vi "FTW-Actor-ConstructExtended.vi"(0 "FTW Actor Instance Type":refnum<class "FTW-ActorInstance.lvclass">, 7 "Actor Instance Configuration":string, 11 "error in":errorcluster) -> (4 "FTW Actor Instance":refnum<class "FTW-ActorInstance.lvclass">, 8 "Subscriber Registration":refnum<event-registration>, 15 "error out":errorcluster)   [LabVIEW 2015, in "FTW-ActorInstance.lvclass"]
uses:
  FTW-ActorInstance.lvclass
  Message/Base/FTW-Message.lvclass
  FTW-ActorInstance.lvclass/FTW-ActorInstance.ctl
  Connector/FTW-ActorConnector.lvclass
  Publisher/FTW-Publisher.lvclass
  Ether/FTW-Ether.lvclass
  Subscriber/FTW-Subscriber.lvclass
panel:
  # "Inputs"
  # "Outputs"
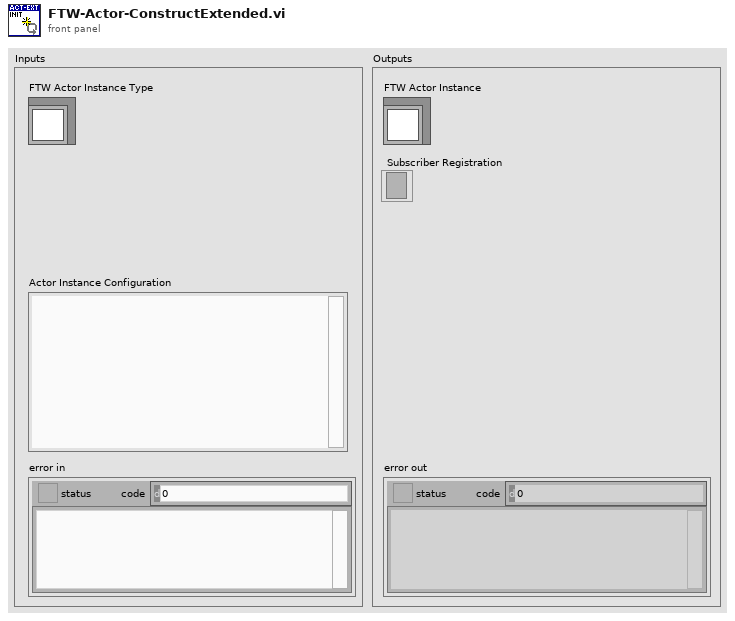
[diagram p1: front panel]
types:
  T1 = cluster{"String":string, "Fetched Address":string, "FTW Actor Connector":refnum<class "FTW-ActorConnector.lvclass">, bool}
  T2 = cluster{"String":string, "Actual Address":string, "FTW-Publisher Out":refnum<class "FTW-Publisher.lvclass">}
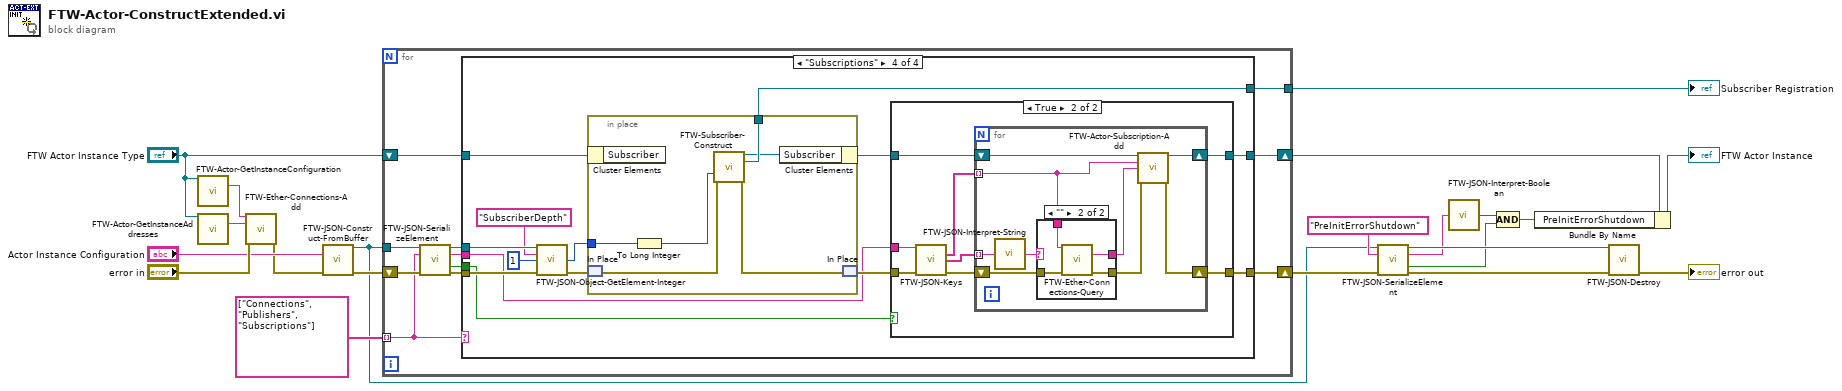
[diagram p0: block diagram]
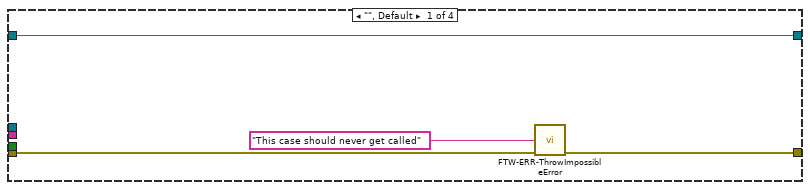
[diagram p2: hidden frame]
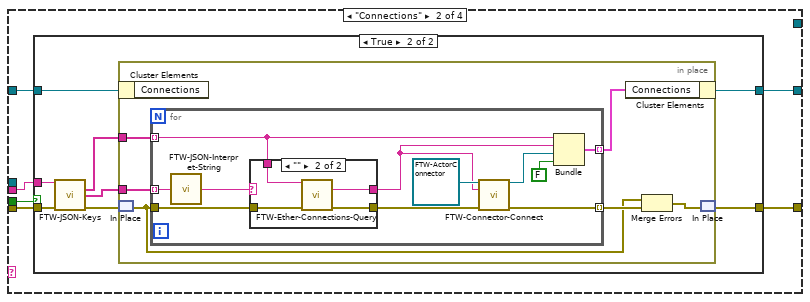
[diagram p3: hidden frame]
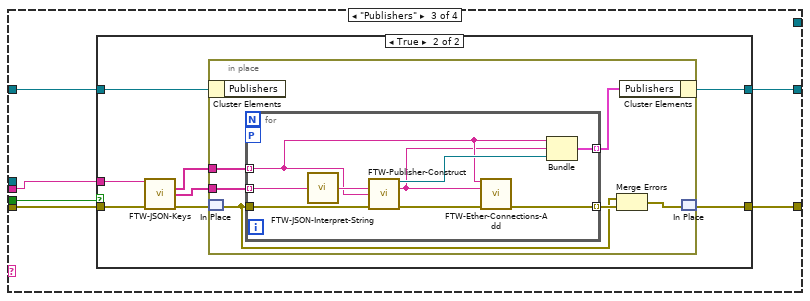
[diagram p6: hidden frame]
diagram:
  n1 = call "FTW-Actor-GetInstanceConfiguration.vi"("FTW Actor Instance"="FTW Actor Instance Type") -> ("Identity"=w4:string)  [unwired: 12 in, 2 out]
  n2 = call "FTW-Actor-GetInstanceAddresses.vi"("FTW Actor Instance"="FTW Actor Instance Type") -> ("Inbox Address"=w3:string)  [unwired: 12 in, 2 out]
  n3 = call "FTW-Ether-Connections-Add.vi"("Connection"=w4, "Address"=w3, "error in"="error in") -> ("error out"=w2:errorcluster)  [unwired: 12 in]
  n4 = call "FTW-JSON-Construct-FromBuffer.vi"("JSON String (UTF-8)"="Actor Instance Configuration", "error in"=w2) -> ("JSON"=w6:refnum<class "FTW-Container.lvclass">, "error out"=w18:errorcluster)  [unwired: 12 in]
  n5 = for {
    tunnel: w6 -> [w32]
    tunnel: string[] ["Connections", "Publishers", "Subscriptions"] -> [w22] mode=indexing
    shift-right: [w27] -> w17
    shift-left: "FTW Actor Instance Type" -> [w28]
    shift-right: [w26] -> w16
    shift-left: w18 -> [w31]
    tunnel: [w25] -> w1
    n6 = call "FTW-JSON-SerializeElement.vi"("JSON"=w32, "Key"=w22, "error in"=w31) -> ("JSON out"=w24:refnum<class "FTW-Container.lvclass">, "Element as JSON String"=w30:string, "Found?"=w23:bool, "error out"=w29:errorcluster)  [unwired: 9 in]
    n7 = case shown="\"Subscriptions\"" w22 {
      tunnel: w30 -> [_ w38 w77 w116]
      tunnel: w29 -> [w35 w40 w79 w119]
      tunnel: w28 -> [w36 w42 w81 w120]
      tunnel: [w36 w41 w80 w113] -> w27
      tunnel: [w34 w39 w78 w115] -> w26
      tunnel: [_ _ _ w117] -> w25
      tunnel: w24 -> [_ _ _ w111]
      tunnel: w23 -> [_ w37 w76 w108]
      frame "", Default {
        n8 = call "FTW-ERR-ThrowImpossibleError.vi"("Reason this error should never happen"="This case should never get called", "error in"=w35) -> ("error out"=w34:errorcluster)  [unwired: 13 in]
      }
      frame "Connections" {
        n9 = case shown="True" w37 {
          tunnel: w42 -> [w44 w52]
          tunnel: [w44 w51] -> w41
          tunnel: w40 -> [w43 w50]
          tunnel: [w43 w46] -> w39
          tunnel: w38 -> [_ w45]
          frame False {
          }
          frame True {
            n10 = call "FTW-JSON-Keys.vi"("JSON Opject"=w45, "error in"=w50) -> ("Keys"=w49:string[], "Values"=w48:string[], "error out"=w47:errorcluster)  [unwired: 11 in]
            n11 = in-place {
              in-place-border: w49 -> [w55]
              in-place-border: w48 -> [w58]
              n12 = in-place-cluster #1(w52) -> ()  [unwired: 1 out]
              n13 = in-place-match #2(w47) -> (w53:errorcluster)
              n14 = for {
                tunnel: w53 -> [w67]
                tunnel: w58 -> [w68] mode=indexing
                tunnel: [w69] -> w57 mode=indexing
                tunnel: w55 -> [w60] mode=indexing
                tunnel: [w64] -> w54 mode=indexing
                n15 = call "FTW-JSON-Interpret-String.vi"("JSON String"=w68) -> ("LabVIEW String"=w61:string)
                n16 = case shown="\"\"" w61 {
                  selector: w61 -> [w71 _]
                  tunnel: w67 -> [w70 w75]
                  tunnel: [w70 w74] -> w62
                  tunnel: w60 -> [_ w73]
                  tunnel: [w71 w72] -> w59
                  frame Default {
                  }
                  frame "" {
                    n17 = call "FTW-Ether-Connections-Query.vi"("Connection"=w73, "error in"=w75) -> ("Fetched Address"=w72:string, "error out"=w74:errorcluster)  [unwired: 12 in]
                  }
                }
                n18 = call-dynamic "FTW-Connector-Connect.vi"("FTW Actor Connector Type"=refnum<class "FTW-ActorConnector.lvclass"> refnum, "Instance Inbox Address"=w59, "error in"=w62) -> ("FTW Actor Connector"=w65:refnum<class "FTW-ActorConnector.lvclass">, "error out"=w69:errorcluster)  [unwired: 11 in]
                n19 = Bundle("String"=w60, "Fetched Address"=w59, "FTW Actor Connector"=w65, FALSE) -> (w64:T1)  [unwired: 1 in]
              }
              n20 = in-place-cluster #1("Connections"=w54) -> (w51:refnum<class "FTW-ActorInstance.lvclass">)
              n21 = Merge Errors(w53, w57) -> (w56:errorcluster)
              n22 = in-place-match #2(w56) -> (w46:errorcluster)
            }
          }
        }
      }
      frame "Publishers" {
        n23 = case shown="True" w76 {
          tunnel: w81 -> [w83 w91]
          tunnel: [w83 w90] -> w80
          tunnel: w79 -> [w82 w89]
          tunnel: [w82 w85] -> w78
          tunnel: w77 -> [_ w84]
          frame False {
          }
          frame True {
            n24 = call "FTW-JSON-Keys.vi"("JSON Opject"=w84, "error in"=w89) -> ("Keys"=w88:string[], "Values"=w87:string[], "error out"=w86:errorcluster)  [unwired: 11 in]
            n25 = in-place {
              in-place-border: w88 -> [w93]
              in-place-border: w87 -> [w97]
              n26 = in-place-cluster #3(w91) -> ()  [unwired: 1 out]
              n27 = in-place-match #4(w86) -> (w92:errorcluster)
              n28 = for {
                tunnel: w92 -> [w105]
                tunnel: w97 -> [w106] mode=indexing
                tunnel: w93 -> [w99] mode=indexing
                tunnel: [w100] -> w96 mode=indexing
                workers-P: _ -> [_]
                tunnel: [w101] -> w94 mode=indexing
                n29 = call "FTW-JSON-Interpret-String.vi"("JSON String"=w106) -> ("LabVIEW String"=w103:string)
                n30 = call "FTW-Publisher-Construct.vi"("Address"=w103, "Identity"=w99, "error in"=w105) -> ("FTW-Publisher Out"=w102:refnum<class "FTW-Publisher.lvclass">, "Actual Address"=w98:string, "error out"=w104:errorcluster)  [unwired: 10 in]
                n31 = call "FTW-Ether-Connections-Add.vi"("Connection"=w99, "Address"=w98, "error in"=w104) -> ("error out"=w100:errorcluster)  [unwired: 12 in]
                n32 = Bundle("String"=w99, "Actual Address"=w98, "FTW-Publisher Out"=w102) -> (w101:T2)  [unwired: 1 in]
              }
              n33 = Merge Errors(w92, w96) -> (w95:errorcluster)
              n34 = in-place-cluster #3("Publishers"=w94) -> (w90:refnum<class "FTW-ActorInstance.lvclass">)
              n35 = in-place-match #4(w95) -> (w85:errorcluster)
            }
          }
        }
      }
      frame "Subscriptions" {
        n36 = call "FTW-JSON-Object-GetElement-Integer.vi"("JSON"=w111, "Key"="SubscriberDepth", "Default Value"=i64 1, "error in"=w119) -> ("Value"=w109:i64, "error out"=w112:errorcluster)  [unwired: 7 in, 3 out]
        n37 = in-place {
          in-place-border: [w149] -> w117
          in-place-border: w109 -> [w147]
          n38 = in-place-cluster #5(w120) -> ()  [unwired: 1 out]
          n39 = in-place-match #6(w112) -> (w151:errorcluster)
          n40 = To Long Integer(number=w147) -> (32bit integer=w146:i32)
          n41 = call "FTW-Subscriber-Construct.vi"("Buffer Depth (1 element)"=w146, "error in"=w151) -> ("FTW-Subscription Out"=w148:refnum<class "FTW-Subscriber.lvclass">, "Subscriber Registration"=w149:refnum<event-registration>, "error out"=w150:errorcluster)  [unwired: 11 in]
          n42 = in-place-cluster #5("Subscriber"=w148) -> (w114:refnum<class "FTW-ActorInstance.lvclass">)
          n43 = in-place-match #6(w150) -> (w118:errorcluster)
        }
        n44 = case shown="True" w108 {
          tunnel: w118 -> [w121 w130]
          tunnel: w116 -> [_ w128]
          tunnel: [w121 w127] -> w115
          tunnel: w114 -> [w122 w126]
          tunnel: [w122 w125] -> w113
          frame False {
          }
          frame True {
            n45 = call "FTW-JSON-Keys.vi"("JSON Opject"=w128, "error in"=w130) -> ("Keys"=w123:string[], "Values"=w124:string[], "error out"=w129:errorcluster)  [unwired: 11 in]
            n46 = for {
              shift-right: [w136] -> w125
              shift-left: w126 -> [w137]
              shift-right: [w138] -> w127
              shift-left: w129 -> [w139]
              tunnel: w124 -> [w135] mode=indexing
              tunnel: w123 -> [w132] mode=indexing
              n47 = call "FTW-JSON-Interpret-String.vi"("JSON String"=w135) -> ("LabVIEW String"=w133:string)
              n48 = case shown="\"\"" w133 {
                selector: w133 -> [w141 _]
                tunnel: w139 -> [w140 w145]
                tunnel: [w140 w144] -> w134
                tunnel: w132 -> [_ w143]
                tunnel: [w141 w142] -> w131
                frame Default {
                }
                frame "" {
                  n49 = call "FTW-Ether-Connections-Query.vi"("Connection"=w143, "error in"=w145) -> ("Fetched Address"=w142:string, "error out"=w144:errorcluster)  [unwired: 12 in]
                }
              }
              n50 = call "FTW-Actor-Subscription-Add.vi"("FTW-ActorInstance In"=w137, "Subscriber Name"=w132, "Subscriber URI"=w131, "error in"=w134) -> ("FTW-ActorInstance Out"=w136:refnum<class "FTW-ActorInstance.lvclass">, "error out"=w138:errorcluster)  [unwired: 10 in]
            }
          }
        }
      }
    }
  }
  "Subscriber Registration" <- w1
  n51 = call "FTW-JSON-SerializeElement.vi"("JSON"=w6, "Key"="PreInitErrorShutdown", "error in"=w16) -> ("JSON out"=w11:refnum<class "FTW-Container.lvclass">, "Element as JSON String"=w9:string, "Found?"=w5:bool, "error out"=w12:errorcluster)  [unwired: 9 in]
  n52 = call "FTW-JSON-Interpret-Boolean.vi"("JSON Boolean"=w9) -> ("LabVIEW Boolean"=w8:bool)
  n53 = Compound Arithmetic op=AND(w8, w5) -> (w7:bool)
  n54 = Bundle By Name(cluster=w17, "PreInitErrorShutdown"=w7) -> (→"FTW Actor Instance":refnum<class "FTW-ActorInstance.lvclass">)
  n55 = call "FTW-JSON-Destroy.vi"("JSON"=w11, "error in"=w12) -> ("error out"=→"error out":errorcluster)  [unwired: 13 in]
